vi "PathBuilder.vi"(0 "Path (String)":string="Files\\Database.csv") -> (1 "Directory indicator:":string, 2 "Path (Path)":path)   [LabVIEW 2019]
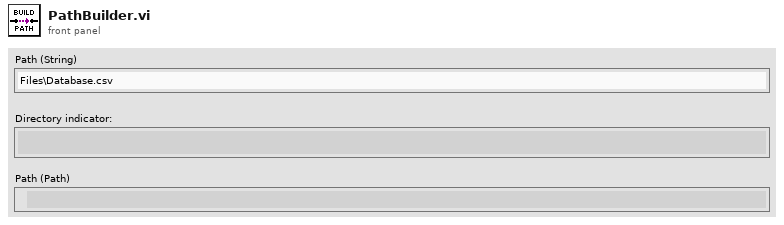
[diagram p1: front panel]
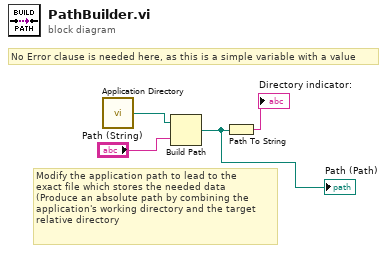
[diagram p0: block diagram]
diagram:
  # "No Error clause is needed here, as this is a simple variable with a value"
  # "Modify the application path to lead to the\nexact file which stores the needed data\n(Produce an absolute path by combining the\napplication's working directory and the target\nrelative directory"
  n1 = call <vilib>:"Application Directory.vi"() -> ("Application Directory"=w4:path)
  n2 = Build Path(base path=w4, name or relative path="Path (String)") -> (appended path=w1:path)
  "Path (Path)" <- w1
  n3 = Path To String(path=w1) -> (string=→"Directory indicator:":string)
